vi "numeric to analog ch enum.vi"(11 "Numeric":i32) -> (3 "Analog Ch":T1)   [LabVIEW 2018]
uses:
  02.Type Def's/EOL Analog Input Control.ctl
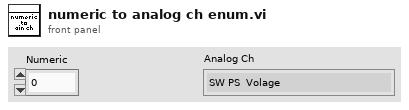
[diagram p1: front panel]
types:
  T1 = typedef "EOL Analog Input Control.ctl" = enum16{"SW PS  Volage", "SW IGN Bat", "Switch A", "Switch B", "Motor Voltage", "Motor Current", "SW LIN", "ATS", "External ECU Current"}
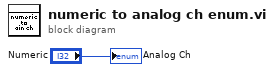
[diagram p0: block diagram]
diagram:
  "Analog Ch" <- "Numeric"
